vi "Get Device Description.vi"(8 "error in (no error)":errorcluster, 10 "Device Index":i32) -> (0 "error out":errorcluster, 2 "Device Description":string)   [LabVIEW 2019, in "D2XX-lv.lvlib"]
doc: "Returns <b>Device Description</b> of device at <b>Device Index</b>."
uses:
  D2XX-lv.lvlib
  <instrlib>/_D2XX/D2XX/D2XX.lvlib
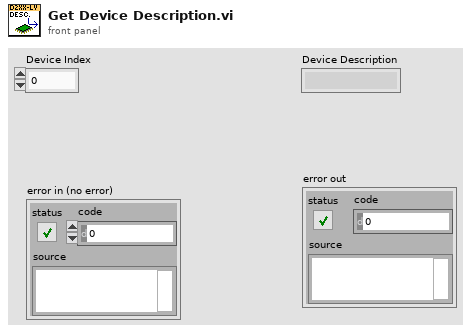
[diagram p1: front panel]
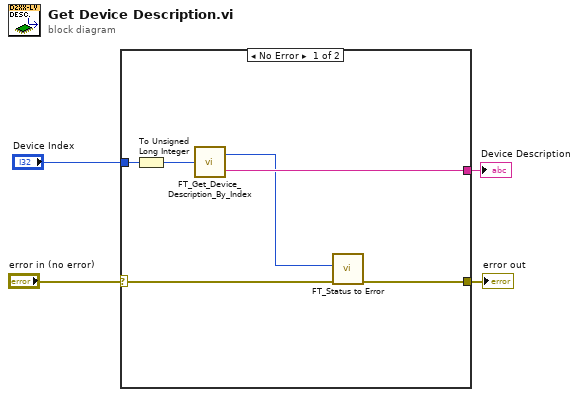
[diagram p0: block diagram]
diagram:
  n1 = case shown="No Error" "error in (no error)" {
    selector: "error in (no error)" -> [w10 w11]
    tunnel: [w9 w11] -> w3
    tunnel: "Device Index" -> [w8 _]
    tunnel: [w7 _] -> w1
    frame No Error {
      n2 = To Unsigned Long Integer(number=w8) -> (unsigned 32bit integer=w5:u32)
      n3 = call <instrlib>:"FT_Get_Device_Description_By_Index.vi"("Device Index"=w5) -> ("FT_Status"=w6:u32, "Device Description"=w7:string)
      n4 = call "FT_Status to Error.vi"("error in (no error)"=w10, "FT_Status"=w6) -> ("error out"=w9:errorcluster)  [unwired: 9 in]
    }
    frame Error {
    }
  }
  "error out" <- w3
  "Device Description" <- w1
